vi "Get MIO.vi"(0 "Session Handle in":T1, 11 "error in (no error)":errorcluster) -> (4 "Session Handle out":T1, 6 "Failure Reason":string, 8 "Failure?":bool, 15 "error out":errorcluster)   [LabVIEW 2014]
uses:
  Typedefs/Session Handle.ctl
  CAN Communicator.lvclass
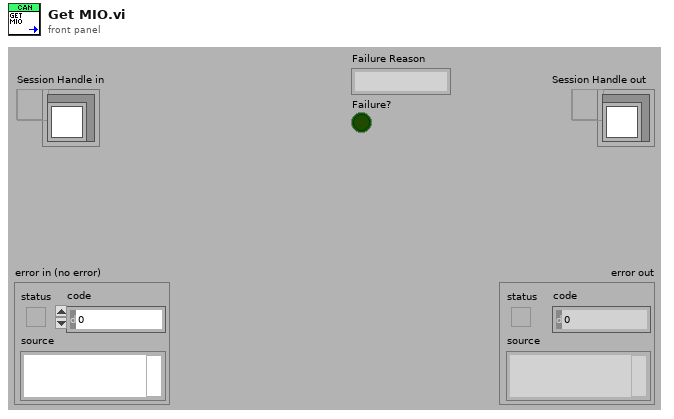
[diagram p1: front panel]
types:
  T1 = typedef "CAN Communicator.lvclass/Session Handle.ctl" = refnum<data-value>
  T2 = typedef "XNET Frame CAN.ctl" = cluster{"timestamp":timestamp, "payload":u8[], "identifier":u32, "type":T3, "extended?":bool, "echo?":bool}
  T3 = typedef "XNET Frame Type CAN.ctl" = u8
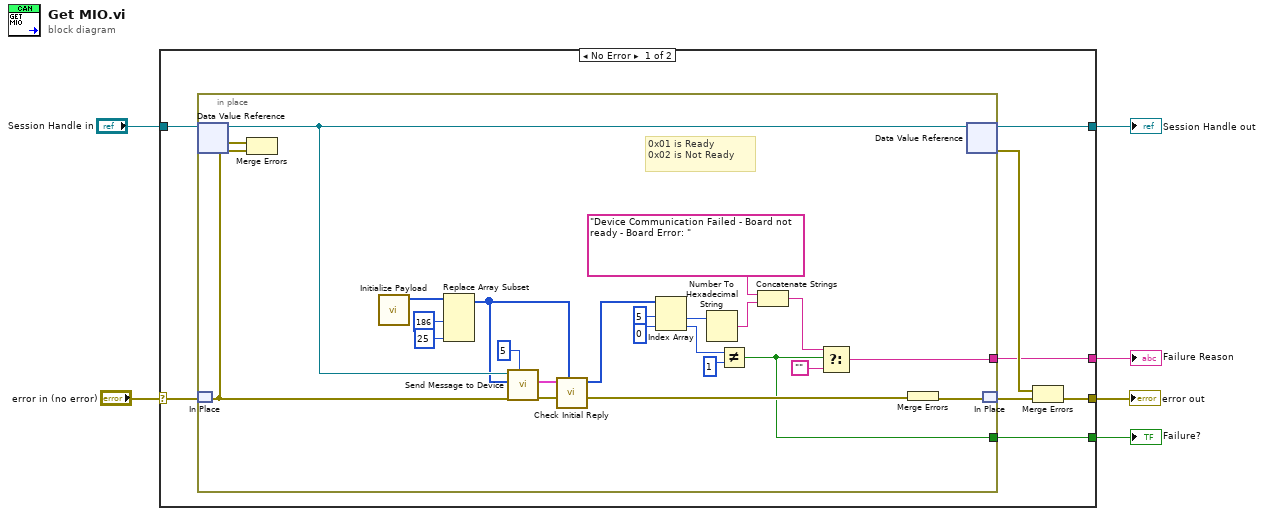
[diagram p0: block diagram]
diagram:
  n1 = case shown="No Error" "error in (no error)" {
    selector: "error in (no error)" -> [w9 w38]
    tunnel: "Session Handle in" -> [w14 w39]
    tunnel: [w13 w39] -> w5
    tunnel: [w10 w38] -> w4
    tunnel: [w8 _] -> w2
    tunnel: [w7 _] -> w1
    frame No Error {
      n2 = in-place {
        in-place-border: [w19] -> w8
        in-place-border: [w15] -> w7
        # "0x01 is Ready\n0x02 is Not Ready"
        n3 = in-place-dvr #1(w14) -> (w36:refnum<class "CAN Communicator.lvclass">, w37:errorcluster)
        n4 = in-place-match #2(w9) -> (w35:errorcluster)
        n5 = Merge Errors(w35, w37) -> ()  [unwired: 1 out]
        n6 = call "Initialize Payload.vi"() -> ("Initial Payload"=w34:u8[])  [unwired: 11 in]
        n7 = Replace Array Subset(array=w34, new element #1=u8 186 ("new element/subarray"), new element #2=u8 25 ("new element/subarray")) -> (w17:u8[])  [unwired: 2 in]
        n8 = call "Send Message to Device.vi"("Number of Retries"=5, "error in (no error)"=w35, "payload"=w17, "CAN Comm In"=w36) -> ("error out"=w24:errorcluster, "Reply"=w18:T2[])  [unwired: 5 in, 1 out]
        n9 = call "Check Initial Reply.vi"("Write Message"=w17, "Reply"=w18) -> ("Data Packet"=w16:u8[])  [unwired: 8 in, 1 out]
        n10 = Index Array(array=w16, index #1=5 ("index"), index #2=0 ("index")) -> (element #1=w27:u8, element #2=w29:u8)
        n11 = Number To Hexadecimal String(2:w27) -> (0:w26:string)  [unwired: 1 in]
        n12 = Not Equal?(x=w29, y=u8 1 ("new element/subarray")) -> (x != y?=w15:bool)
        n13 = Concatenate Strings("Device Communication Failed - Board not ready - Board Error: " ("string"), w26) -> (w20:string)
        n14 = Select(t=w20, s=w15, f="") -> (s? t:f=w19:string)
        n15 = Merge Errors(w24) -> (w23:errorcluster)
        n16 = in-place-dvr #1(w36) -> (w13:T1, w11:errorcluster)
        n17 = in-place-match #2(w23) -> (w12:errorcluster)
      }
      n18 = Merge Errors(w11, w12) -> (w10:errorcluster)
    }
    frame Error {
    }
  }
  "Session Handle out" <- w5
  "error out" <- w4
  "Failure Reason" <- w2
  "Failure?" <- w1
